vi "InitializeNetworkStreamReader.vi"() -> (0 "error out":errorcluster, 3 "NetworkStreamReader out":refnum<class "NetworkStreamReader.lvclass">)   [LabVIEW 2013]
doc: "Initializes the network stream reader."
uses:
  RIO-OCU_Comm/NetworkStreams/Reader/NetworkStreamReader.lvclass
  Location of Think.ctl
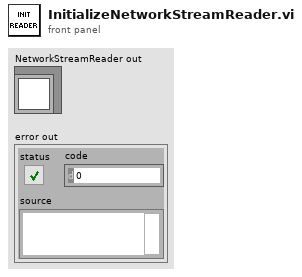
[diagram p1: front panel]
types:
  T1 = typedef "Location of Think.ctl" = string
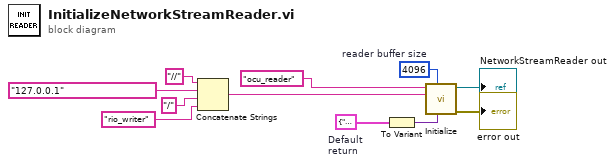
[diagram p0: block diagram]
diagram:
  w8 = cluster{"Name":string, "value":variant} {"Name"="", "value"=variant}  # Default return
  w5 = 4096  # reader buffer size
  n1 = Concatenate Strings("//" ("string"), T1 "127.0.0.1" ("Location of THINK"), "/", "rio_writer" ("string")) -> (w7:string)
  n2 = To Variant(anything=w8) -> (Variant=w9:variant)
  n3 = call "Initialize.vi"("Default return"=w9, "reader buffer size"=w5, "writer url"=w7, "reader name"="ocu_reader" ("writer name")) -> ("error out"=→"error out":errorcluster, "NetworkStreamReader out"=→"NetworkStreamReader out":refnum<class "NetworkStreamReader.lvclass">)  [unwired: 6 in]
